vi "to.cluster_pairs.vi"(8 "error in":errorcluster, 11 "properties in":refnum<class "properties.lvclass">) -> (0 "error out":errorcluster, 2 "Properties":cluster{"name":string, "value":string}[](array[cluster]), 3 "properties out":refnum<class "properties.lvclass">)   [LabVIEW 2020, in "nominal types.lvlib" / "properties.lvclass"]
uses:
  properties.lvclass
  properties.lvclass/properties.ctl
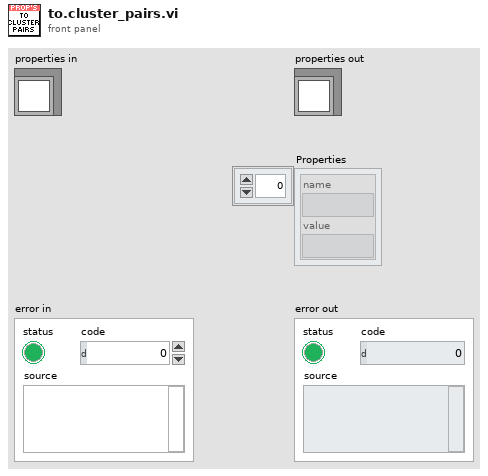
[diagram p1: front panel]
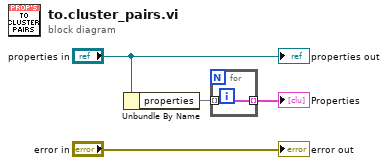
[diagram p0: block diagram]
diagram:
  n1 = Unbundle By Name("properties in") -> ("properties"=w2:map{string, string})
  n2 = for {
    tunnel: w2 -> [w5] mode=indexing
    tunnel: [w5] -> w1 mode=indexing
  }
  "Properties" <- w1
  "properties out" <- "properties in"
  "error out" <- "error in"
